vi "Initialize.vi"(8 "error in":errorcluster, 10 "Device":string) -> (0 "error out":errorcluster, 3 "Laser out":refnum<class "Laser.lvclass">)   [LabVIEW 2018, in "Laser.lvlib" / "Laser.lvclass"]
uses:
  Laser.lvclass
  Laser.lvclass/Laser.ctl
  PPLs/Configuration/Configuration.lvlibp/Configuration.lvclass
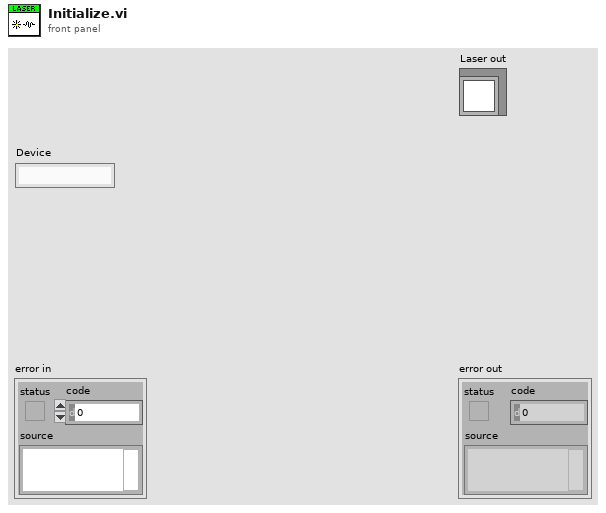
[diagram p1: front panel]
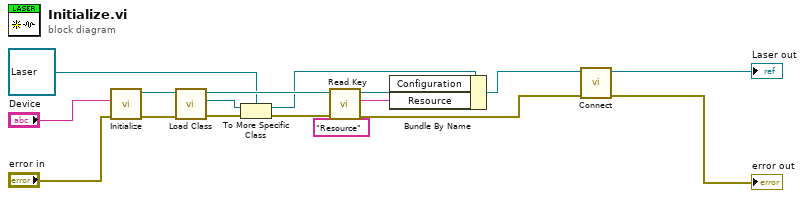
[diagram p0: block diagram]
diagram:
  n1 = call "Initialize.vi"("error in"="error in", "Device"="Device") -> ("error out"=w7:errorcluster, "Configuration out"=w17:refnum<class "Configuration.lvclass">)  [unwired: 8 in]
  n2 = call "Load Class.vi"("error in"=w7, "Configuration in"=w17) -> ("error out"=w14:errorcluster, "Class out"=w15:refnum<class>, "Configuration out"=w16:refnum<class "Configuration.lvclass">)  [unwired: 7 in]
  n3 = To More Specific Class(target class=refnum<class "Laser.lvclass"> refnum ("Laser in"), reference=w15, error in=w14) -> (specific class reference=w11:refnum<class "Laser.lvclass">, error out=w13:errorcluster)
  n4 = call "Read Key.vi"("Key:"="Resource", "error in"=w13, "Configuration in"=w16) -> ("error out"=w4:errorcluster, "Value"=w9:string, "Configuration out"=w10:refnum<class "Configuration.lvclass">)  [unwired: 6 in]
  n5 = Bundle By Name(cluster=w11, "Configuration"=w10, "Resource"=w9) -> (w8:refnum<class "Laser.lvclass">)
  n6 = call-dynamic "Connect.vi"("error in (no error)"=w4, "Laser in"=w8) -> ("error out"=→"error out":errorcluster, "Laser out"=→"Laser out":refnum<class "Laser.lvclass">)  [unwired: 8 in]
